vi "UiCharts_b2g1.vi"() -> ()   [LabVIEW 2011]
uses:
  Output - Cluster b2g1.ctl
  Input - Cluster b2g1.ctl
  DBSqlSelectToArray(2DArrayString).vi
panel:
  in  "Output Var":refnum<k21>="ni.var.psp://10.27.40.24/variables - b2g1/data - network - b2g1"
  in  "Input Var":refnum<k21>="ni.var.psp://10.27.40.24/variables - b2g1/input - network b2g1"
  in  "Tab Control":T1(tab)
  out "protocol":string[][](table)
  out "pH-Wert":dbl(graph)
  out "Temperaturregelung MR":T2(graph)
  out "Temperaturregelung T-3":T3(graph)
  out "Füllstandsregelung":T4(graph)
  out "Druckregelung":T5(graph)
  in  "plant":enum16{"B2G1", "B2G2"}(ring)
  in  "sensor":T6(ring)
  in  "begin":timestamp=timestamp(3427135200 s since 1904-01-01) format="%<%X\n%x>T"
  in  "end":timestamp=timestamp(3427221599.999 s since 1904-01-01) format="%<%X\n%x>T"
  in  "load":bool
  out "XY Graph":cluster{timestamp, dbl}[](graph)
  out "error out":errorcluster
  in  "stop":bool
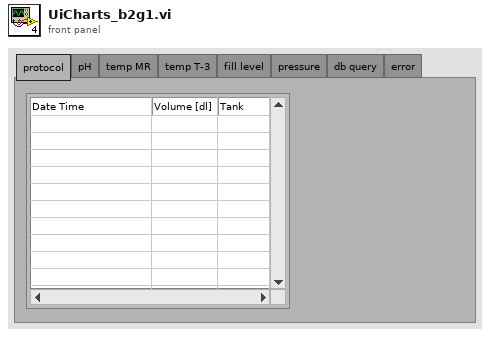
[diagram p1: front panel]
types:
  T1 = enum32{"protocol", "pH", "temp MR", "temp T-3", "fill level", "pressure", "db query", "error"}
  T2 = cluster{"Temp Soll MR [°C]":sgl, "TS-4 [°C]":dbl, "TS-5 [°C]":dbl, dbl, dbl}
  T3 = cluster{"Temp Soll T-3 [°C] 2":sgl, "TS-6 [°C]":dbl, dbl, sgl}
  T4 = cluster{"Füllstand Soll [l]":sgl, "FS-3 [l]":dbl, dbl}
  T5 = cluster{"Druck Soll [bar]":sgl, "DS-1 [bar]":dbl, dbl, dbl}
  T6 = enum16{"pressure", "temperature 4", "temperature 5", "pH-value", "fill level 1", "fill level 2", "fill level 3"}
  T7 = typedef "Input - Cluster b2g1.ctl" = cluster{"Log-Target":bool, "P-4":bool, "P-4 Drehzahl [%]":u8, "Temperaturregelung MR":bool, "Überdruckregelung":bool, "Füllstandsregulierung":bool, "Log-Host":bool, "P-5":bool, "P-5 Drehzahl [%]":u8, "HS-1":bool, "Füllstand  P":sgl, "Füllstand I":sgl, "Füllstand D":sgl, "Füllstand Soll [l]":sgl, "Druck  P":sgl, "Druck I":sgl, "Druck D":sgl, "Druck Soll [bar]":sgl, "Temp Soll MR [°C]":sgl, "Hysterese MR [°C]":sgl, "Log Target [ms]":u32, "Log Host [s]":u32, "P-9":bool, "HS-2":bool, "V-13 [%]":u8, "V-15 [%]":u8, "V-10":bool, "V-14":bool, "Dosierung":bool, "Dosiermenge [l]":sgl, "Dosiergeschw. [l/min]":sgl, "Tank":bool, "MR Füllstandsüberwachung":bool, "Tank Füllstandsüberwachung":bool, "P-5 EIN [min]":u8, "P-5 AUS [min]":u8, "Zirkulation":bool, "V-33":bool, "V-34":bool, "Temperaturregelung T-3":bool, "Temp Soll T-3 [°C] 2":sgl, "Hysterese T-3 [°C] 2":sgl}
  T8 = typedef "Output - Cluster b2g1.ctl" = cluster{"DFS-1 [dl]":u64, "FS-3 [l]":dbl, "DFS-1 [l/min]":dbl, "DS-1 [bar]":dbl, "V-10 ZU":bool, "V-14 ZU":bool, "FS-1 [l]":dbl, "FS-2 [l]":dbl, "TS-4 [°C]":dbl, "HS-1":bool, "V-13 [%]":u8, "V-15 [%]":u8, "P-4 [%]":u8, "P-5 [%]":u8, "Dosierung":bool, "MR Max Füllstand":bool, "MR Min Füllstand":bool, "Dosiermenge [l]":sgl, "V-14 AUF":bool, "V-10 AUF":bool, "T-1 Max Füllstand":bool, "T-1 Min Füllstand":bool, "T-2 Max Füllstand":bool, "T-2 Min Füllstand":bool, "pHS-1 [pH]":dbl, "P-4 RUN":bool, "P-5 RUN ":bool, "V-33 AUF":bool, "V-33 ZU":bool, "V-34 AUF":bool, "V-34 ZU":bool, "P-4 ERR":bool, "P-5 ERR":bool, "TS-5 [°C]":dbl, "TS-6 [°C]":dbl, "P-9 RUN":bool, "HS-2":bool}
  T9 = cluster{"Temp Soll MR [°C]":sgl, "TS-4 [°C]":dbl, dbl, dbl, "TS-5 [°C]":dbl}
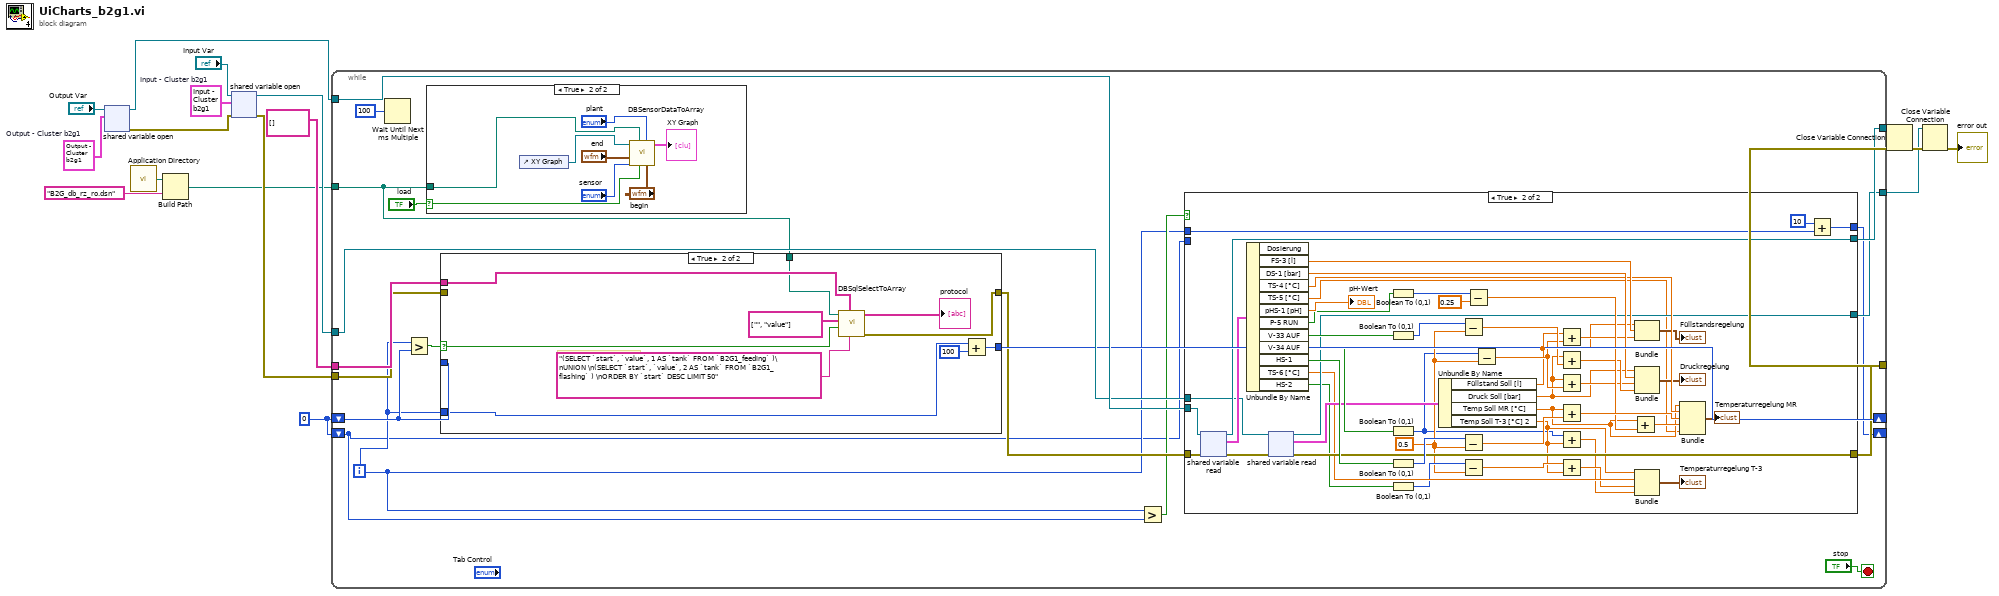
[diagram p0: block diagram]
diagram:
  w14 = T7 {"Log-Target"=FALSE, "P-4"=FALSE, "P-4 Drehzahl [%]"=0, "Temperaturregelung MR"=FALSE, "Überdruckregelung"=FALSE, "Füllstandsregulierung"=FALSE, "Log-Host"=FALSE, "P-5"=FALSE, "P-5 Drehzahl [%]"=0, "HS-1"=FALSE, "Füllstand  P"=0.0, "Füllstand I"=0.0, "Füllstand D"=0.0, "Füllstand Soll [l]"=0.0, "Druck  P"=0.0, "Druck I"=0.0, "Druck D"=0.0, "Druck Soll [bar]"=0.0, "Temp Soll MR [°C]"=0.0, "Hysterese MR [°C]"=0.0, "Log Target [ms]"=0, "Log Host [s]"=0, "P-9"=FALSE, "HS-2"=FALSE, "V-13 [%]"=0, "V-15 [%]"=0, "V-10"=FALSE, "V-14"=FALSE, "Dosierung"=FALSE, "Dosiermenge [l]"=0.0, "Dosiergeschw. [l/min]"=0.0, "Tank"=FALSE, "MR Füllstandsüberwachung"=FALSE, "Tank Füllstandsüberwachung"=FALSE, "P-5 EIN [min]"=0, "P-5 AUS [min]"=0, "Zirkulation"=FALSE, "V-33"=FALSE, "V-34"=FALSE, "Temperaturregelung T-3"=FALSE, "Temp Soll T-3 [°C] 2"=0.0, "Hysterese T-3 [°C] 2"=0.0}  # Input - Cluster b2g1
  w17 = T8 {"DFS-1 [dl]"=0, "FS-3 [l]"=0.0, "DFS-1 [l/min]"=0.0, "DS-1 [bar]"=0.0, "V-10 ZU"=FALSE, "V-14 ZU"=FALSE, "FS-1 [l]"=0.0, "FS-2 [l]"=0.0, "TS-4 [°C]"=0.0, "HS-1"=FALSE, "V-13 [%]"=0, "V-15 [%]"=0, "P-4 [%]"=0, "P-5 [%]"=0, "Dosierung"=FALSE, "MR Max Füllstand"=FALSE, "MR Min Füllstand"=FALSE, "Dosiermenge [l]"=0.0, "V-14 AUF"=FALSE, "V-10 AUF"=FALSE, "T-1 Max Füllstand"=FALSE, "T-1 Min Füllstand"=FALSE, "T-2 Max Füllstand"=FALSE, "T-2 Min Füllstand"=FALSE, "pHS-1 [pH]"=0.0, "P-4 RUN"=FALSE, "P-5 RUN "=FALSE, "V-33 AUF"=FALSE, "V-33 ZU"=FALSE, "V-34 AUF"=FALSE, "V-34 ZU"=FALSE, "P-4 ERR"=FALSE, "P-5 ERR"=FALSE, "TS-5 [°C]"=0.0, "TS-6 [°C]"=0.0, "P-9 RUN"=FALSE, "HS-2"=FALSE}  # Output - Cluster b2g1
  w4 = u32 0
  n1 = shared-variable-open("Output Var", w17) -> (w16:refnum<k21>, w11:errorcluster)  [unwired: 2 in]
  n2 = call <vilib>:"Application Directory.vi"() -> ("Application Directory"=w3:path)
  n3 = Build Path(base path=w3, name or relative path="B2G_db_rz_ro.dsn" ("Name of ini file 2")) -> (appended path=w1:path)
  n4 = shared-variable-open("Input Var", w11, w14) -> (w12:refnum<k21>, w6:errorcluster)  [unwired: 1 in]
  n5 = while {
    tunnel: w16 -> [w37]
    tunnel: [w36] -> w15
    tunnel: w12 -> [w35]
    tunnel: [w34] -> w9
    tunnel: string[][] [] ("data") -> [w33]
    shift-right: [w31] -> _
    shift-left: w4 -> [w24]
    tunnel: w6 -> [w28]
    tunnel: [w27] -> w5
    shift-right: [w22] -> _
    shift-left: w4 -> [w21]
    tunnel: w1 -> [w19]
    i -> [w23]
    stop <- "stop" stop-if-true
    n6 = Wait Until Next ms Multiple(millisecond multiple=100) -> ()  [unwired: 1 out]
    n7 = Greater?(x=w23, y=w24) -> (0:w32:bool)
    n8 = case shown="True" "load" {
      selector: "load" -> [_ w39]
      tunnel: w19 -> [_ w38]
      frame False {
      }
      frame True {
        n9 = control-ref of="XY Graph"() -> (w41:refnum<vi>)
        n10 = call "DBSensorDataToArray.vi"("begin"="begin", "plant"="plant", "load"=w39, "appended path"=w38, "sensor"="sensor", "end"="end", "XYGraph in"=w41) -> ("shift reg out"=→"XY Graph":cluster{timestamp, dbl}[])  [unwired: 3 in, 1 out]
      }
    }
    n11 = case shown="True" w32 {
      selector: w32 -> [_ w104]
      tunnel: [w101 w110] -> w31
      tunnel: w24 -> [w101 _]
      tunnel: w23 -> [_ w111]
      tunnel: w33 -> [_ w107]
      tunnel: w28 -> [w100 _]
      tunnel: [w100 w106] -> w29
      tunnel: w19 -> [_ w102]
      frame False {
      }
      frame True {
        # "WHERE `value` > 0"
        n12 = call-poly "DBSqlSelectToArray.vi"("String"="(SELECT `start`, `value`, 1 AS `tank` FROM `B2G1_feeding` )\nUNION \n(SELECT `start`, `value`, 2 AS `tank` FROM `B2G1_flashing` ) \nORDER BY `start` DESC LIMIT 50" ("SQL query"), "shift reg in"=w107, "enable"=w104, "format"=string[][] [["", "value"]] ("columns"), "connection information"=w102) -> ("error out"=w106:errorcluster, "shift reg out"=→"protocol":string[][])  [unwired: 5 in]
        n13 = Add(x=w111, y=i64 100) -> (x+y=w110:i64)
      }
    }
    n14 = Greater?(x=w23, y=w21) -> (0:w25:bool)
    n15 = case shown="True" w25 {
      tunnel: w37 -> [w47 w99]
      tunnel: [w47 w98] -> w36
      tunnel: w29 -> [w49 w75]
      tunnel: [w49 w73] -> w27
      tunnel: w35 -> [w48 w72]
      tunnel: [w48 w67] -> w34
      tunnel: w23 -> [_ w66]
      tunnel: [w46 w64] -> w22
      tunnel: w21 -> [w46 _]
      frame False {
      }
      frame True {
        w55 = 0.5 ("y")
        n16 = shared-variable-read(w99, w75) -> (w98:refnum<k21>, w74:errorcluster, w97:T8)  [unwired: 1 out]
        n17 = Unbundle By Name(w97) -> ("FS-3 [l]"=w96:dbl, "DS-1 [bar]"=w95:dbl, "TS-4 [°C]"=w94:dbl, "TS-5 [°C]"=w61:dbl, "pHS-1 [pH]"=→"pH-Wert":dbl, "P-5 RUN"=w90:bool, "V-33 AUF"=w92:bool, "V-34 AUF"=w91:bool, "HS-1"=w89:bool, "TS-6 [°C]"=w58:dbl, "HS-2"=w56:bool)  [unwired: 1 out]
        n18 = shared-variable-read(w72, w74) -> (w67:refnum<k21>, w73:errorcluster, w71:T7)  [unwired: 1 out]
        n19 = Boolean To (0,1)(Boolean=w90) -> (0, 1=w83:i16)
        n20 = Boolean To (0,1)(Boolean=w92) -> (0, 1=w76:i16)
        n21 = Boolean To (0,1)(Boolean=w91) -> (0, 1=w50:i16)
        n22 = Boolean To (0,1)(Boolean=w89) -> (0, 1=w86:i16)
        n23 = Boolean To (0,1)(Boolean=w56) -> (0, 1=w57:i16)
        n24 = Unbundle By Name(w71) -> ("Füllstand Soll [l]"=w70:sgl, "Druck Soll [bar]"=w68:sgl, "Temp Soll MR [°C]"=w69:sgl, "Temp Soll T-3 [°C] 2"=w52:sgl)
        n25 = Subtract(x=w76, y=w55) -> (x-y=w81:dbl)
        n26 = Subtract(x=w86, y=w55) -> (x-y=w88:dbl)
        n27 = Subtract(x=w57, y=w55) -> (x-y=w54:dbl)
        n28 = Subtract(x=w83, y=0.25) -> (x-y=w85:dbl)
        n29 = Subtract(x=w50, y=w55) -> (x-y=w77:dbl)
        n30 = Add(x=w70, y=w77) -> (x+y=w78:dbl)
        n31 = Add(x=w68, y=w81) -> (x+y=w80:dbl)
        n32 = Add(x=w68, y=w77) -> (x+y=w79:dbl)
        n33 = Add(x=w69, y=w88) -> (x+y=w87:dbl)
        n34 = Add(x=w50, y=w52) -> (x+y=w51:sgl)
        n35 = Add(x=w54, y=w52) -> (x+y=w53:dbl)
        n36 = Add(x=w69, y=w85) -> (x+y=w82:dbl)
        n37 = Bundle("Füllstand Soll [l]"=w70, "FS-3 [l]"=w96, w78) -> (→"Füllstandsregelung":T4)  [unwired: 1 in]
        n38 = Bundle("Druck Soll [bar]"=w68, "DS-1 [bar]"=w95, w79, w80) -> (→"Druckregelung":T5)  [unwired: 1 in]
        n39 = Bundle("Temp Soll T-3 [°C] 2"=w52, "TS-6 [°C]"=w58, w53, w51) -> (→"Temperaturregelung T-3":T3)  [unwired: 1 in]
        n40 = Bundle("Temp Soll MR [°C]"=w69, "TS-4 [°C]"=w94, w87, w82, "TS-5 [°C]"=w61) -> (→"Temperaturregelung MR":T9)  [unwired: 1 in]
        n41 = Add(x=10, y=w66) -> (x+y=w64:i32)
      }
    }
  }
  n42 = Close Variable Connection(8:w5, 11:w15) -> (0:w10:errorcluster)
  n43 = Close Variable Connection(8:w10, 11:w9) -> (0:→"error out":errorcluster)
